vi "Multipples_posiciones.vi"(0 "Pasos por vuelta\nM1                 M2              M3            M4":dbl[](array[numeric]), 4 "Directorio scripts matlab 2":path=path "C:/Users/franjas/Documents/rutinas-calibracion-slm", 6 "File Path Control":path=path "C:/Users/franjas/Documents/rutinas-calibracion-slm/measures.txt", 9 "Seleción método":bool, 11 "Nombre de archivo 2":string="In1") -> (1 "?":bool, 8 "subarray":dbl[](array[numeric]))   [LabVIEW 2013]
uses:
  <vilib>/Analysis/Matrix/Datatypes/RealMatrix.ctl
  <vilib>/Utility/file.llb/Read From Spreadsheet File (DBL).vi
  <vilib>/Analysis/Matrix/NI_Matrix.lvlib
panel:
  out "Real Matrix":T1
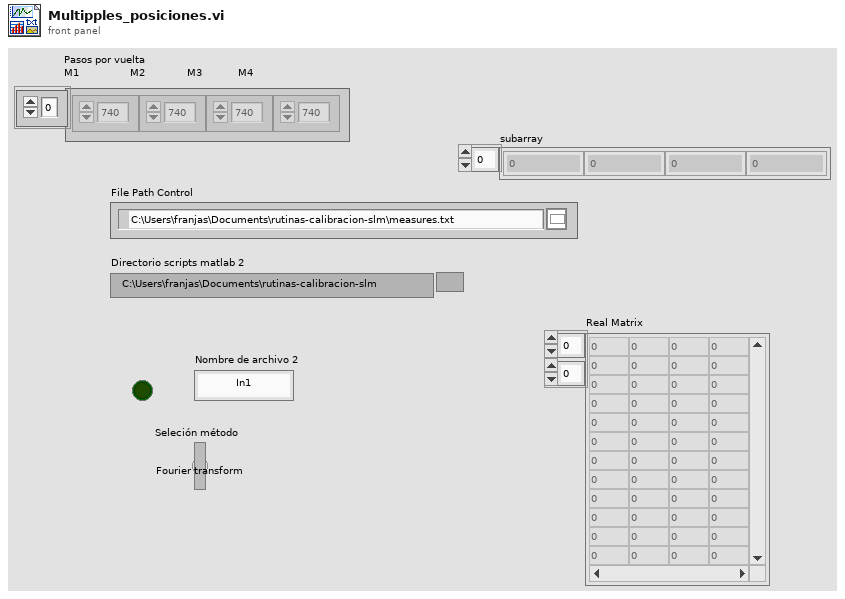
[diagram p1: front panel]
types:
  T1 = typedef "NI_Matrix.lvlib/RealMatrix.ctl" = dbl[][]
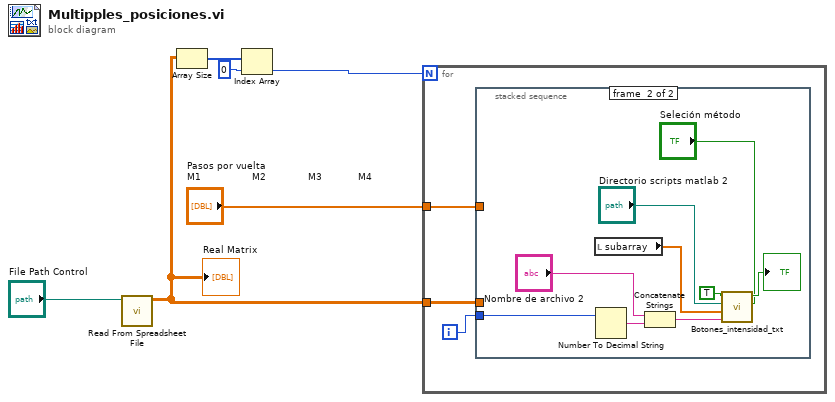
[diagram p0: block diagram]
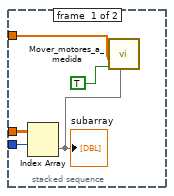
[diagram p2: hidden frame]
diagram:
  n1 = call-poly <vilib>:"Read From Spreadsheet File.vi"("file path (dialog if empty)"="File Path Control") -> ("all rows"=w2:dbl[][])  [unwired: 6 in, 4 out]
  "Real Matrix" <- w2
  n2 = Array Size(array=w2) -> (size(s)=w5:i32[])
  n3 = Index Array(array=w5, index=0) -> (element=w3:i32)
  n4 = for {
    N: w3 -> [_]
    tunnel: w2 -> [w9]
    tunnel: "Pasos por vuelta\nM1                 M2              M3            M4" -> [w7]
    i -> [w8]
    n5 = stacked-sequence {
      tunnel: w9 -> [w12 _]
      tunnel: w8 -> [w11 w21]
      tunnel: w7 -> [w10 _]
      frame #0 {
        n6 = Index Array(array=w12, index (row)=w11) -> (element=w14:dbl[])  [unwired: 1 in]
        "subarray" <- w14
        n7 = call "Mover_motores_a_medida.vi"("Ángulos de elementos ópticos:\nL2_in          L4_in        L4_out     P__out 2"=w14, "Run"=TRUE ("Boolean"), "Pasos por vuelta\nM1                 M2              M3            M4"=w10) -> ()  [unwired: 9 in]
      }
      frame #1 {
        n8 = local read "subarray"() -> (w15:dbl[])
        n9 = Number To Decimal String(number=w21) -> (decimal integer string=w18:string)  [unwired: 1 in]
        n10 = Concatenate Strings("Nombre de archivo 2", w18) -> (w19:string)
        n11 = call "Botones_intensidad_txt.vi"("Seleción método"="Seleción método", "String"=w19, "Array"=w15, "Directorio scripts matlab 2"="Directorio scripts matlab 2", "I1"=TRUE) -> (3:→"?":bool)  [unwired: 6 in]
      }
    }
  }
